vi "MakeScreenshot.vi"(5 "type screenshot":enum16{"graph", "window"}(ring), 6 "Compress the picture?":bool, 7 "Visible area only? (f)":bool, 8 "error in (no error)":errorcluster, 9 "String in":refnum<vi>, 10 "XYGraph Refnum":refnum<vi>, 11 "VI in":refnum<vi>) -> (0 "error out":errorcluster, 2 "Image path":path)   [LabVIEW 2018]
doc: "This example captures an image of the front panel of a VI and saves the image to a JPG, PNG, or BMP file."
uses:
  <vilib>/wsapi/NI_WebServices.lvlib
panel:
  out "Base64 String":string
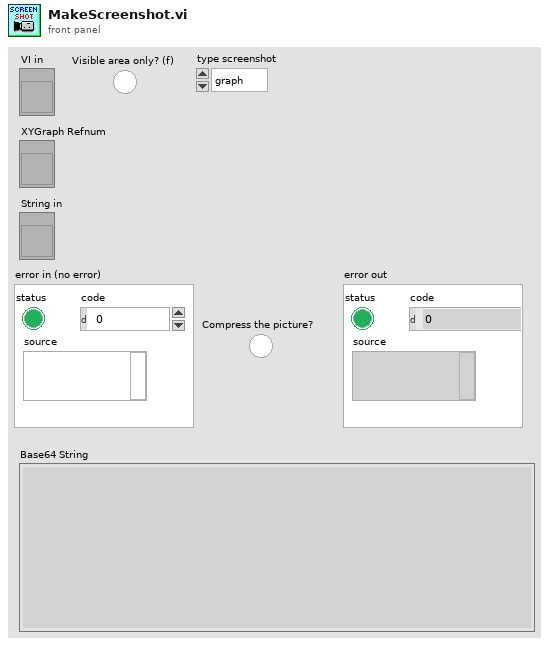
[diagram p1: front panel]
types:
  T1 = typedef "imagedata.ctl" = cluster{"image type":i32, "image depth":i32, "image":u8[], "mask":u8[], "colors":u32[], "Rectangle":cluster{"left":i16, "top":i16, "right":i16, "bottom":i16}}
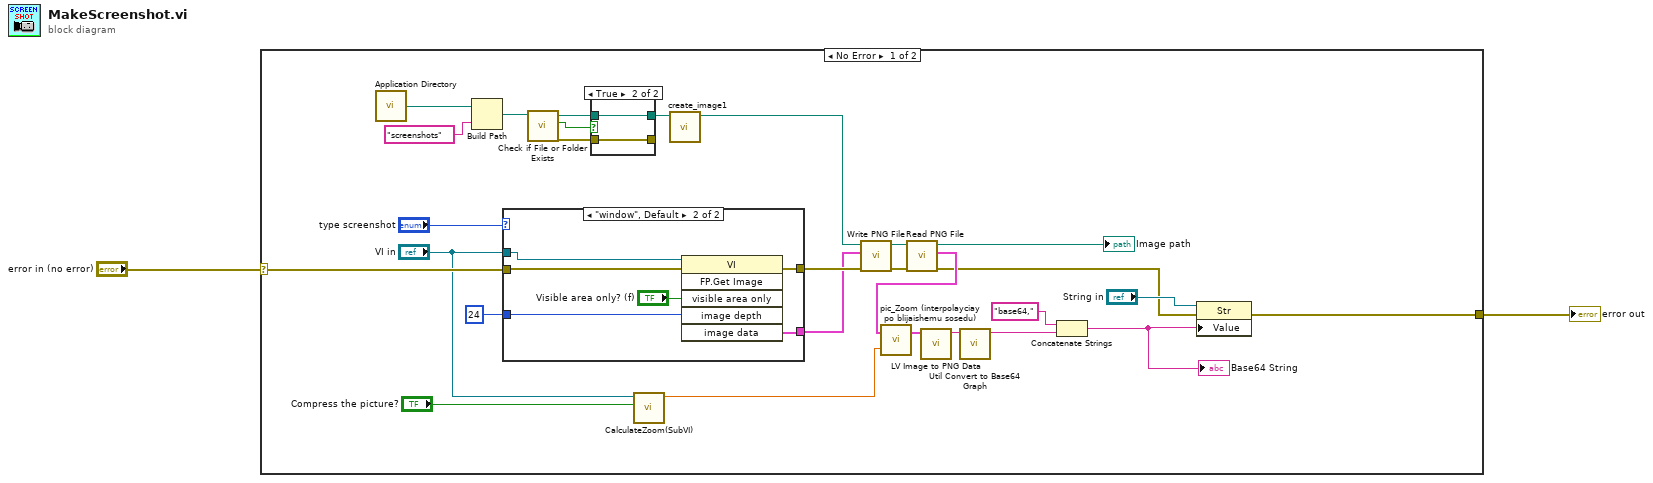
[diagram p0: block diagram]
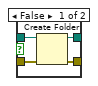
[diagram p2: hidden frame]
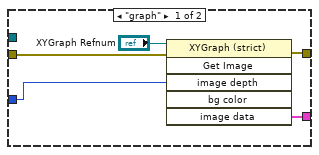
[diagram p3: hidden frame]
diagram:
  n1 = case shown="No Error" "error in (no error)" {
    selector: "error in (no error)" -> [w30 w48]
    tunnel: [w27 w48] -> w2
    frame No Error {
      n2 = call <vilib>:"Application Directory.vi"() -> ("Application Directory"=w22:path)
      n3 = Build Path(base path=w22, name or relative path="screenshots") -> (appended path=w18:path)
      n4 = case shown="\"window\", Default" "type screenshot" {
        tunnel: w30 -> [w39 w47]
        tunnel: [w40 w45] -> w24
        tunnel: [w38 w44] -> w26
        tunnel: u32 24 ("Background Color") -> [w37 w43]
        tunnel: "VI in" -> [_ w42]
        frame "graph" {
          n5 = invoke class="XYGraph (strict)" method="Get Image"(reference="XYGraph Refnum", error in=w39, "image depth"=w37) -> (error out=w38:errorcluster, "image data"=w40:T1)  [unwired: 3 in, 4 out]
        }
        frame "window", Default {
          n6 = invoke class="VI" method="FP.Get Image"(reference=w42, error in=w47, "visible area only"="Visible area only? (f)", "image depth"=w43) -> (error out=w44:errorcluster, "image data"=w45:T1)  [unwired: 2 in, 4 out]
        }
      }
      n7 = call <vilib>:"Check if File or Folder Exists.vi"("path"=w18) -> ("error out"=w19:errorcluster, "file or folder exists?"=w21:bool, "dup path"=w20:path)  [unwired: 8 in]
      n8 = case shown="True" w21 {
        tunnel: w20 -> [w34 w35]
        tunnel: w19 -> [w33 w36]
        tunnel: [w32 w36] -> _
        tunnel: [w31 w35] -> w17
        frame False {
          n9 = Create Folder(path (use dialog)=w34, error in=w33) -> (created path=w31:path, error out=w32:errorcluster)  [unwired: 1 in, 1 out]
        }
        frame True {
        }
      }
      n10 = call "CalculateZoom(SubVI).vi"("Compress the picture?"="Compress the picture?", "VI in"="VI in") -> ("Zoom"=w11:dbl)  [unwired: 9 in]
      n11 = call "create_image1.vi"("base path"=w17) -> ("path"=w28:path)  [unwired: 9 in, 1 out]
      n12 = call <vilib>:"Write PNG File.vi"("error in (no error)"=w26, "image data"=w24, "path to PNG file"=w28) -> ("error out"=w13:errorcluster, "path"=w16:path)  [unwired: 7 in]
      n13 = call <vilib>:"Read PNG File.vi"("error in (no error)"=w13, "path to PNG file"=w16) -> ("error out"=w3:errorcluster, "image data"=w14:T1, "path"=→"Image path":path)  [unwired: 7 in]
      n14 = call "pic_Zoom (interpolayciay po blijaishemu sosedu).vi"("Zoom"=w11, "image data IN"=w14) -> ("image data OUT"=w8:T1)  [unwired: 1 in]
      n15 = call <vilib>:"LV Image to PNG Data.vi"("image data"=w8) -> ("png data"=w7:string)  [unwired: 9 in, 1 out]
      n16 = call "Util Convert to Base64 Graph.vi"("String"=w7) -> ("Base64 String"=w5:string)  [unwired: 10 in]
      n17 = Concatenate Strings("base64," ("string"), w5) -> (w4:string)
      "Base64 String" <- w4
      n18 = property on="Property Node" class="Str"(reference="String in", error in=w3, "Value"=w4) -> (error out=w27:errorcluster)  [unwired: 1 out]
    }
    frame Error {
    }
  }
  "error out" <- w2
